vi "Inputs.vi"(8 "error in (no error)":errorcluster, 11 "Node Ptr":T1 format="%.0x") -> (0 "error out":errorcluster)   [LabVIEW 2015, in "Diagnostics Addon System Explorer.lvlib"]
uses:
  Diagnostics Addon System Explorer.lvlib
  <vilib>/NI Veristand/Custom Device API/Custom Device Item Ref.ctl
  Shared/FG Action.ctl
  Shared/GUID Lookup.vi
  <vilib>/NI Veristand/Custom Device API/NI VeriStand - Set Item Property.vi
  <vilib>/NI Veristand/Custom Device API/Set Item Property (U32).vi
  <vilib>/NI Veristand/Custom Device API/NI VeriStand - Get Item Property.vi
  <vilib>/NI Veristand/Custom Device API/Get Item Property (U32).vi
  <vilib>/NI Veristand/Custom Device API/Custom Device API.lvlib
  Shared/Diagnostics Addon Shared.lvlib
panel:
  in  "SHDocVw.IWebBrowser":refnum<k7>(container)
  in  "PIDs":i32(listbox)
  in  "Description":string
  out "Name":string
  in  "Header":cluster{"Section Name":string}={"Section Name"="Custom Device Item Settings"}
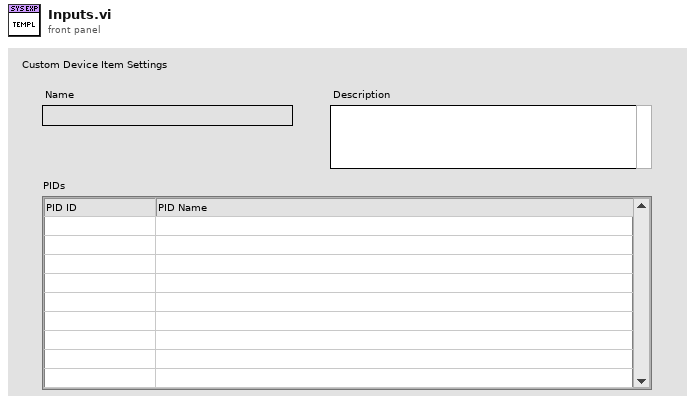
[diagram p1: front panel]
types:
  T1 = typedef "Custom Device API.lvlib/Custom Device Item Ref.ctl" = u64
  T2 = typedef "Diagnostics Addon Shared.lvlib/FG Action.ctl" = enum16{"Get", "Set"}
  T3 = typedef "Custom Device API.lvlib/Custom Device Item Info.ctl" = cluster{"Name":string, "Is Channel":bool, "GUID":string, "Is Waveform":bool}
  T4 = typedef "Custom Device API.lvlib/Custom Device Commands.ctl" = enum16{"Default", "Item renamed", "Shutdown", "Dynamic button pressed"}
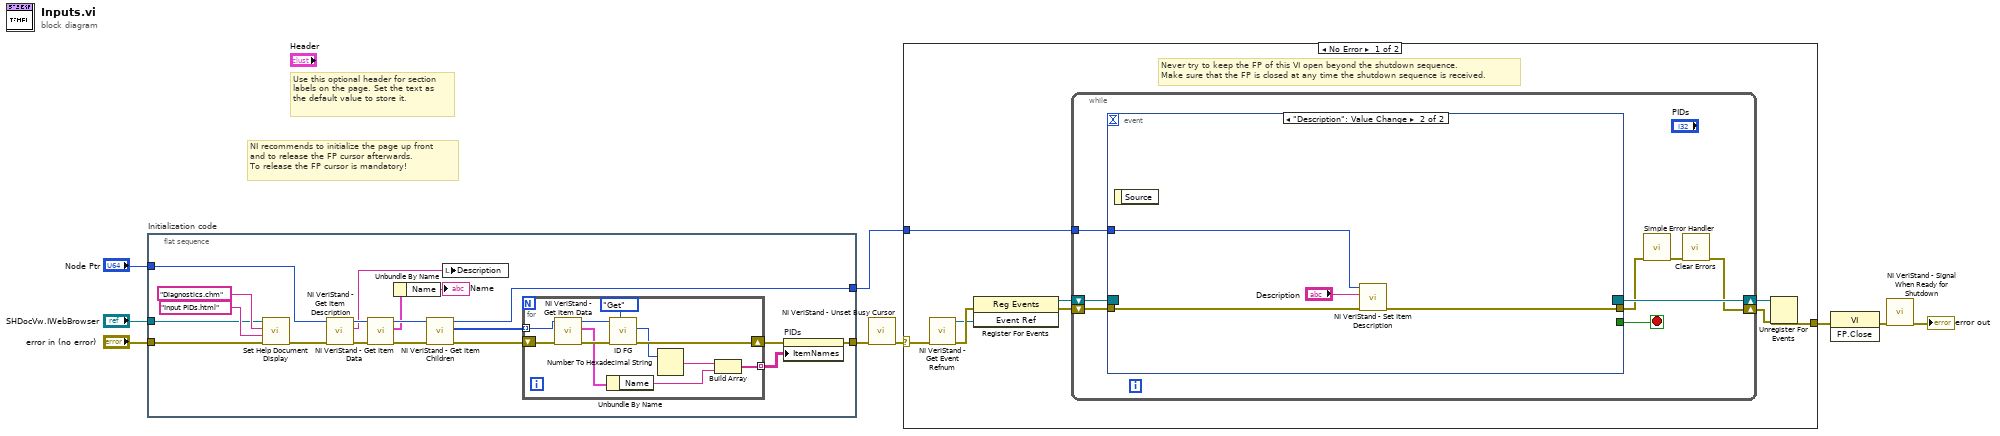
[diagram p0: block diagram]
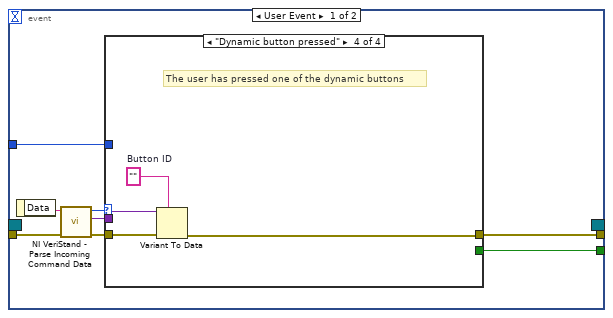
[diagram p2: hidden frame]
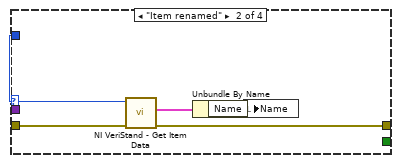
[diagram p4: hidden frame]
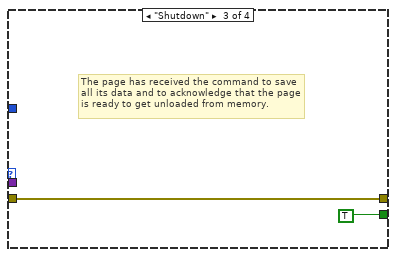
[diagram p5: hidden frame]
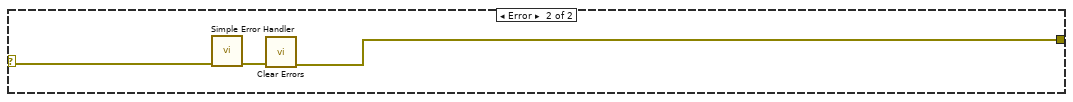
[diagram p6: hidden frame]
diagram:
  # "Use this optional header for section labels on the page. Set the text as the default value to store it."
  # "NI recommends to initialize the page up front\nand to release the FP cursor afterwards.\nTo release the FP cursor is mandatory!"
  n1 = flat-sequence "Initialization code" {
    tunnel: "error in (no error)" -> [w21]
    tunnel: [w12] -> w6
    tunnel: [w14] -> w3
    tunnel: "Node Ptr" -> [w19]
    tunnel: "SHDocVw.IWebBrowser" -> [w18]
    frame #0 {
      n2 = call "Set Help Document Display.vi"("error in (no error)"=w21, "HTML File"="Input PIDs.html", "Main CHM File"="Diagnostics.chm", "SHDocVw.IWebBrowser2"=w18) -> ("error out"=w20:errorcluster)  [unwired: 7 in]
      n3 = call <vilib>:"NI VeriStand - Get Item Description.vi"("error in (no error)"=w20, "Item Ref in"=w19) -> ("error out"=w25:errorcluster, "Description"=w26:string, "Item Ref out"=w27:T1)  [unwired: 7 out]
      n4 = call <vilib>:"NI VeriStand - Get Item Data.vi"("error in (no error)"=w25, "Item Ref in"=w27) -> ("error out"=w17:errorcluster, "Item Info"=w24:T3, "Item Ref out"=w28:T1)  [unwired: 7 out]
      n5 = Unbundle By Name(w24) -> ("Name"=→"Name":string)
      n6 = call <vilib>:"NI VeriStand - Get Item Children.vi"("error in (no error)"=w17, "Item Ref in"=w28) -> ("error out"=w16:errorcluster, "Child Refs"=w15:T1[], "Item Ref out"=w14:T1)  [unwired: 6 in, 1 out]
      n7 = local write "Description"(w26) -> ()
      n8 = for {
        shift-right: [w35] -> w13
        shift-left: w16 -> [w39]
        tunnel: w15 -> [w38] mode=indexing
        tunnel: [w30] -> w11 mode=indexing
        n9 = call <vilib>:"NI VeriStand - Get Item Data.vi"("error in (no error)"=w39, "Item Ref in"=w38) -> ("error out"=w37:errorcluster, "Item Info"=w34:T3, "Item Ref out"=w36:T1)  [unwired: 7 out]
        n10 = Unbundle By Name(w34) -> ("Name"=w31:string)
        n11 = call "ID FG.vi"("Action"=FG_Action."Get", "error in (no error)"=w37, "Device Item Ref in"=w36) -> ("error out"=w35:errorcluster, "ID"=w33:u32)  [unwired: 6 in, 1 out]
        n12 = Number To Hexadecimal String(2:w33) -> (0:w32:string)  [unwired: 1 in]
        n13 = Build Array(w32, w31) -> (w30:string[])
      }
      n14 = property on="PIDs" class="MCListbox (strict)"(error in=w13, "ItemNames"=w11) -> (error out=w12:errorcluster)  [unwired: 1 in, 1 out]
    }
  }
  n15 = call <vilib>:"NI VeriStand - Unset Busy Cursor.vi"("error in (no error)"=w6) -> ("error out"=w5:errorcluster)  [unwired: 10 out]
  n16 = case shown="No Error" w5 {
    selector: w5 -> [w40 w83]
    tunnel: [w45 w81] -> w9
    tunnel: w3 -> [w41 _]
    frame No Error {
      # "Never try to keep the FP of this VI open beyond the shutdown sequence.\nMake sure that the FP is closed at any time the shutdown sequence is received."
      n17 = call <vilib>:"NI VeriStand - Get Event Refnum.vi"("error in (no error)"=w40) -> ("error out"=w48:errorcluster, "Event Ref"=w44:refnum<user-event>)  [unwired: 9 out]
      n18 = register-events(error in=w48, w44) -> (reference out=w42:refnum<event-registration>, error out=w43:errorcluster)  [unwired: 1 in]
      n19 = while {
        tunnel: w41 -> [w52]
        shift-right: [w49] -> w46
        shift-left: w43 -> [w55]
        shift-right: [w56] -> w47
        shift-left: w42 -> [w54]
        stop <- w53 stop-if-true
        n20 = event shown="[1] \"Description\": Value Change" {
          selector: w54 -> [_ _]
          dyn-events: [_ _] -> w56
          timeout: _ -> [_ _]
          tunnel: w55 -> [w64 w79]
          tunnel: [w60 _] -> w53
          tunnel: [w59 w78] -> w51
          tunnel: w52 -> [w58 w80]
          event User Event {
            n21 = event-data() -> ("Data"=w63:string)  [unwired: 1 out]
            n22 = call <vilib>:"NI VeriStand - Parse Incoming Command Data.vi"("error in (no error)"=w64, "Incoming data"=w63) -> ("error out"=w62:errorcluster, "Outgoing data"=w57:variant, "Action"=w61:T4)  [unwired: 7 out]
            n23 = case shown="\"Dynamic button pressed\"" w61 {
              tunnel: w62 -> [w65 w70 w71 w76]
              tunnel: [_ _ TRUE _] -> w60
              tunnel: [w65 w67 w71 w73] -> w59
              tunnel: w58 -> [_ w69 _ _]
              tunnel: w57 -> [_ _ _ w75]
              frame "Default", Default {
              }
              frame "Item renamed" {
                n24 = call <vilib>:"NI VeriStand - Get Item Data.vi"("error in (no error)"=w70, "Item Ref in"=w69) -> ("error out"=w67:errorcluster, "Item Info"=w68:T3)  [unwired: 8 out]
                n25 = Unbundle By Name(w68) -> ("Name"=w66:string)
                n26 = local write "Name"(w66) -> ()
              }
              frame "Shutdown" {
                # "The page has received the command to save all its data and to acknowledge that the page is ready to get unloaded from memory."
              }
              frame "Dynamic button pressed" {
                w74 = ""  # Button ID
                # "The user has pressed one of the dynamic buttons"
                n27 = Variant To Data(error in=w76, type=w74, Variant=w75) -> (error out=w73:errorcluster)  [unwired: 1 out]
              }
            }
          }
          event "Description": Value Change {
            n28 = event-data() -> ()  [unwired: 2 out]
            n29 = call <vilib>:"NI VeriStand - Set Item Description.vi"("error in (no error)"=w79, "Description"="Description", "Item Ref in"=w80) -> ("error out"=w78:errorcluster)  [unwired: 8 out]
          }
        }
        n30 = call <vilib>:"Simple Error Handler.vi"("error in (no error)"=w51) -> ("error out"=w50:errorcluster)  [unwired: 1 in, 7 out]
        n31 = call <vilib>:"Clear Errors.vi"("error in (no error)"=w50) -> ("error out"=w49:errorcluster)  [unwired: 1 in, 5 out]
      }
      n32 = Unregister For Events(event registration refnum=w47, error in=w46) -> (error out=w45:errorcluster)
    }
    frame Error {
      n33 = call <vilib>:"Simple Error Handler.vi"("error in (no error)"=w83) -> ("error out"=w82:errorcluster)  [unwired: 1 in, 7 out]
      n34 = call <vilib>:"Clear Errors.vi"("error in (no error)"=w82) -> ("error out"=w81:errorcluster)  [unwired: 1 in, 5 out]
    }
  }
  n35 = invoke class="VI" method="FP.Close"(error in=w9) -> (error out=w8:errorcluster)  [unwired: 2 in, 2 out]
  n36 = call <vilib>:"NI VeriStand - Signal When Ready for Shutdown.vi"("error in (no error)"=w8) -> ("error out"=→"error out":errorcluster)  [unwired: 10 out]
